vi "test2.vi"() -> ()   [LabVIEW 2018]
uses:
  Socket/Socket.lvclass
  <vilib>/addons/zeromq/socket_type.ctl
  <vilib>/addons/zeromq/zeromq.lvlib
panel:
  out "error out":errorcluster
  in  "Socket in":refnum<class "Socket.lvclass">
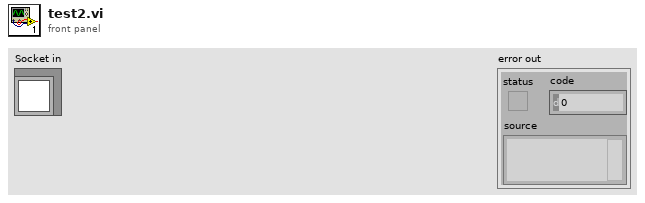
[diagram p1: front panel]
types:
  T1 = typedef "zeromq.lvlib/socket_type.ctl" = enum8{"ZMQ_PAIR", "ZMQ_PUB", "ZMQ_SUB", "ZMQ_REQ", "ZMQ_REP", "ZMQ_DEALER", "ZMQ_ROUTER", "ZMQ_PULL", "ZMQ_PUSH", "ZMQ_XPUB", "ZMQ_XSUB", "ZMQ_STREAM", "ZMQ_SERVER", "ZMQ_CLIENT", "ZMQ_RADIO", "ZMQ_DISH", "ZMQ_GATHER", "ZMQ_SCATTER", "ZMQ_DGRAM"}
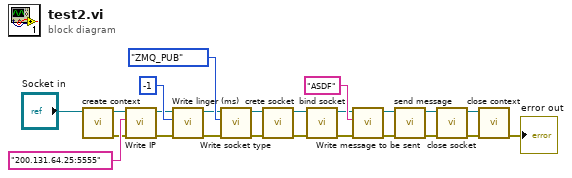
[diagram p0: block diagram]
diagram:
  n1 = call "create context.vi"("Socket in"="Socket in") -> ("error out"=w1:errorcluster, "Socket out"=w6:refnum<class "Socket.lvclass">)  [unwired: 9 in]
  n2 = call-dynamic "Write IP.vi"("error in (no error)"=w1, "IP"="200.131.64.25:5555", "Socket in"=w6) -> ("error out"=w20:errorcluster, "Socket out"=w17:refnum<class "Socket.lvclass">)  [unwired: 7 in]
  n3 = call-dynamic "Write linger (ms).vi"("error in (no error)"=w20, "linger (ms)"=-1, "Socket in"=w17) -> ("error out"=w19:errorcluster, "Socket out"=w18:refnum<class "Socket.lvclass">)  [unwired: 7 in]
  n4 = call-dynamic "Write socket type.vi"("error in (no error)"=w19, "Socket type"=socket_type."ZMQ_PUB", "Socket in"=w18) -> ("error out"=w8:errorcluster, "Socket out"=w9:refnum<class "Socket.lvclass">)  [unwired: 7 in]
  n5 = call "crete socket.vi"("error in (no error)"=w8, "Socket in"=w9) -> ("error out"=w15:errorcluster, "Socket out"=w16:refnum<class "Socket.lvclass">)  [unwired: 8 in]
  n6 = call "bind socket.vi"("error in (no error)"=w15, "Socket in"=w16) -> ("error out"=w4:errorcluster, "Socket out"=w5:refnum<class "Socket.lvclass">)  [unwired: 8 in]
  n7 = call-dynamic "Write message to be sent.vi"("error in (no error)"=w4, "message to be sent"="ASDF", "Socket in"=w5) -> ("error out"=w14:errorcluster, "Socket out"=w11:refnum<class "Socket.lvclass">)  [unwired: 7 in]
  n8 = call "send message.vi"("error in (no error)"=w14, "Socket in"=w11) -> ("error out"=w13:errorcluster, "Socket out"=w12:refnum<class "Socket.lvclass">)  [unwired: 8 in]
  n9 = call "close socket.vi"("error in (no error)"=w13, "Socket in"=w12) -> ("error out"=w2:errorcluster, "Socket out"=w3:refnum<class "Socket.lvclass">)  [unwired: 8 in]
  n10 = call-dynamic "close context.vi"("error in (no error)"=w2, "Socket in"=w3) -> ("error out"=→"error out":errorcluster)  [unwired: 8 in, 1 out]
